vi "WriteTestItem.vi"() -> ()   [LabVIEW 2013]
panel:
  out "error out":errorcluster caption="错误输出"
  in  "error in":errorcluster caption="错误输入（无错误）"
  out "输出数组":string[](array[string])
  out "连接的字符串":string
  out "ReportStrA":string
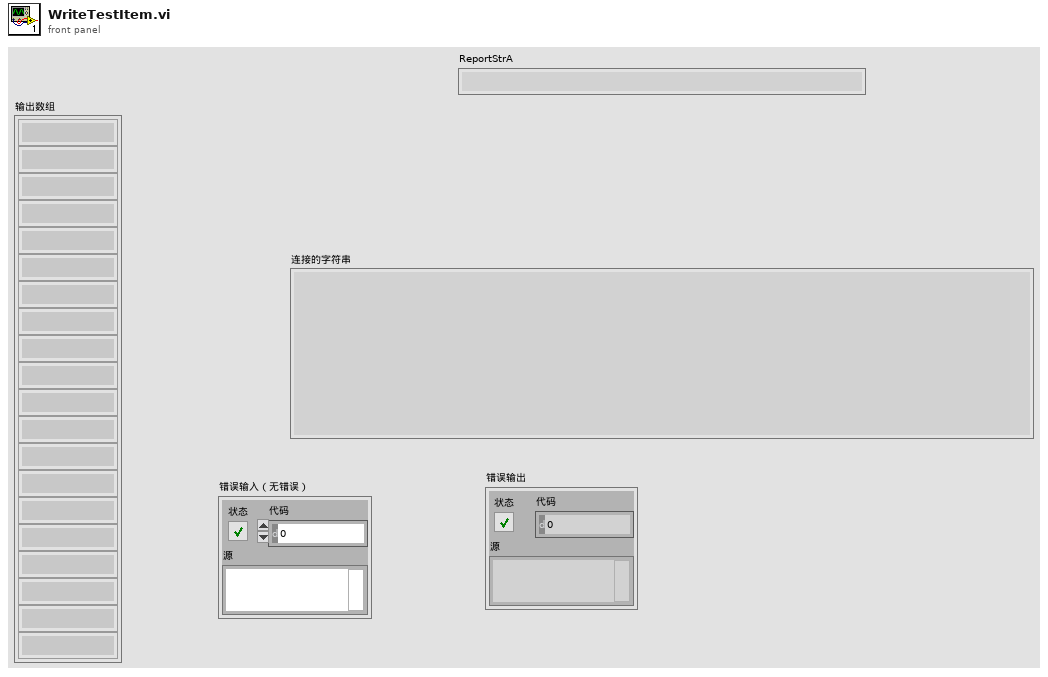
[diagram p1: front panel]
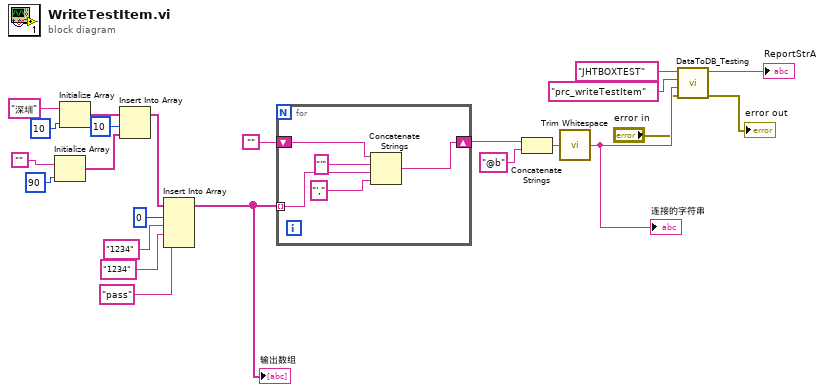
[diagram p0: block diagram]
diagram:
  n1 = Initialize Array("", 90 ("维数大小")) -> (w1:string[])
  n2 = Initialize Array("深圳", 10 ("维数大小")) -> (w6:string[])
  n3 = Insert Into Array(array=w6, index=10 ("索引"), new element=w1) -> (w5:string[])
  n4 = Insert Into Array(array=w5, index=0 ("索引"), new element #1="1234", new element #2="1234", new element #3="pass") -> (w11:string[])
  "输出数组" <- w11
  n5 = for {
    shift-right: [w24] -> w15
    shift-left: "" -> [w28]
    tunnel: w11 -> [w25] mode=indexing
    n6 = Concatenate Strings(w28, "'", w25, "',") -> (w24:string)
  }
  n7 = Concatenate Strings(w15, "@b") -> (w13:string)
  n8 = call <vilib>:"Trim Whitespace.vi"("string"=w13) -> ("trimmed string"=w12:string)  [unwired: 1 in]
  "连接的字符串" <- w12
  n9 = call "DataToDB_Testing.vi"("error in (no error)"="error in", "all string"=w12, "Procedure name"="prc_writeTestItem", "DSN name"="JHTBOXTEST") -> ("error out"=→"error out":errorcluster, "ReportStrA"=→"ReportStrA":string)  [unwired: 6 in]
